vi "out1.vi"() -> ()   [LabVIEW 2018]
panel:
  in  "stop":bool
  in  "amp":dbl(slide) scale=0.0..10.0
  in  "freq":dbl(slide) scale=0.0..500.0
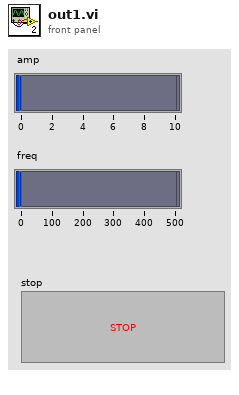
[diagram p1: front panel]
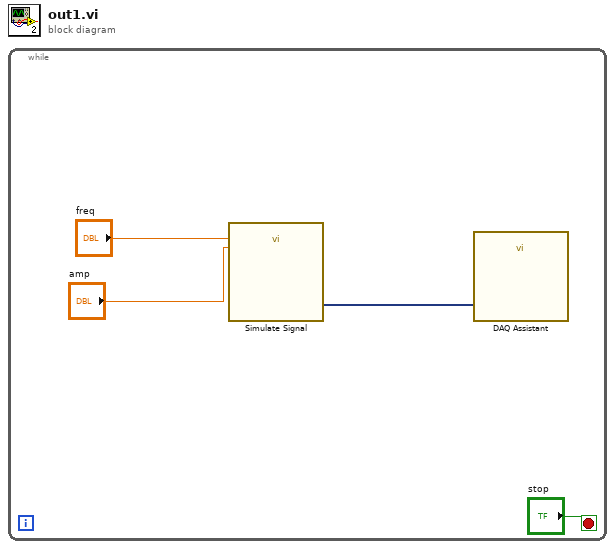
[diagram p0: block diagram]
diagram:
  n1 = while {
    stop <- "stop" stop-if-true
    n2 = call "Simulate Signal"("Frequency"="freq", "Amplitude"="amp") -> ("Sine"=w4:dynamicdata)  [unwired: 12 in, 1 out]
    n3 = call "DAQ Assistant"("data"=w4) -> ()  [unwired: 16 in, 3 out]
  }
